vi "Choose Elevator Idle Position.vi"(7 "Hold Low?":bool, 8 "Idle Mode":T1, 10 "Has Trashcan?":bool, 11 "Presets":T2) -> (3 "Pos Out":sgl)   [LabVIEW 2014]
uses:
  Common Code/Elevator Presets.ctl
  Common Code/Elevator Idle Mode.ctl
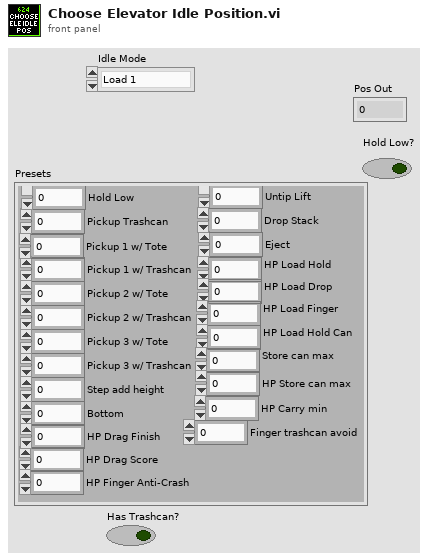
[diagram p1: front panel]
types:
  T1 = typedef "Elevator Idle Mode.ctl" = enum16{"Load 1", "Load 2", "Load 3", "Load Can", "Untip Can", "Step Load", "Drop Stack"}
  T2 = typedef "Elevator Presets.ctl" = cluster{"Pickup 2 w/ Tote":sgl, "Pickup 2 w/ Trashcan":sgl, "Pickup 3 w/ Tote":sgl, "Pickup 3 w/ Trashcan":sgl, "Bottom":sgl, "Pickup 1 w/ Tote":sgl, "Pickup Trashcan":sgl, "Pickup 1 w/ Trashcan":sgl, "Eject":sgl, "Hold Low":sgl, "Step add height":sgl, "Untip Lift":dbl, "Drop Stack":dbl, "HP Load Hold":dbl, "HP Load Drop":dbl, "HP Load Finger":dbl, "HP Load Hold Can":dbl, "Store can max":dbl, "HP Drag Score":dbl, "HP Store can max":dbl, "HP Drag Finish":dbl, "HP Carry min":dbl, "HP Finger Anti-Crash":dbl, "Finger trashcan avoid":dbl}
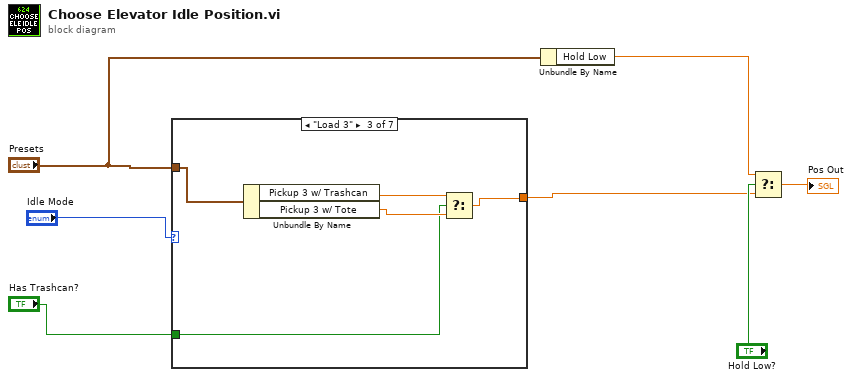
[diagram p0: block diagram]
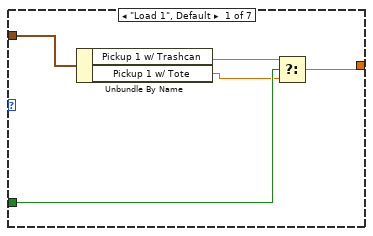
[diagram p2: hidden frame]
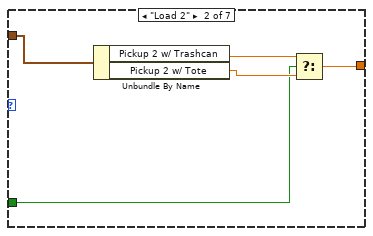
[diagram p3: hidden frame]
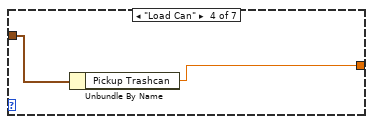
[diagram p4: hidden frame]
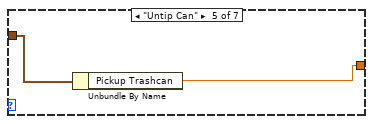
[diagram p5: hidden frame]
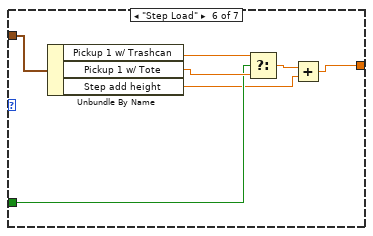
[diagram p6: hidden frame]
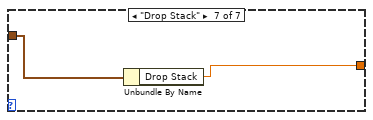
[diagram p7: hidden frame]
diagram:
  n1 = case shown="\"Load 3\"" "Idle Mode" {
    tunnel: "Presets" -> [w12 w14 w18 w24 w26 w31 w35]
    tunnel: "Has Trashcan?" -> [w11 w15 w19 _ _ w30 _]
    tunnel: [w8 w13 w20 w23 w25 w27 w34] -> w1
    frame "Load 1", Default {
      n2 = Unbundle By Name(w12) -> ("Pickup 1 w/ Trashcan"=w10:sgl, "Pickup 1 w/ Tote"=w9:sgl)
      n3 = Select(t=w10, s=w11, f=w9) -> (s? t:f=w8:sgl)
    }
    frame "Load 2" {
      n4 = Unbundle By Name(w14) -> ("Pickup 2 w/ Trashcan"=w17:sgl, "Pickup 2 w/ Tote"=w16:sgl)
      n5 = Select(t=w17, s=w15, f=w16) -> (s? t:f=w13:sgl)
    }
    frame "Load 3" {
      n6 = Unbundle By Name(w18) -> ("Pickup 3 w/ Trashcan"=w21:sgl, "Pickup 3 w/ Tote"=w22:sgl)
      n7 = Select(t=w21, s=w19, f=w22) -> (s? t:f=w20:sgl)
    }
    frame "Load Can" {
      n8 = Unbundle By Name(w24) -> ("Pickup Trashcan"=w23:sgl)
    }
    frame "Untip Can" {
      n9 = Unbundle By Name(w26) -> ("Pickup Trashcan"=w25:sgl)
    }
    frame "Step Load" {
      n10 = Unbundle By Name(w31) -> ("Pickup 1 w/ Trashcan"=w33:sgl, "Pickup 1 w/ Tote"=w32:sgl, "Step add height"=w28:sgl)
      n11 = Select(t=w33, s=w30, f=w32) -> (s? t:f=w29:sgl)
      n12 = Add(x=w29, y=w28) -> (x+y=w27:sgl)
    }
    frame "Drop Stack" {
      n13 = Unbundle By Name(w35) -> ("Drop Stack"=w34:dbl)
    }
  }
  n14 = Unbundle By Name("Presets") -> ("Hold Low"=w6:sgl)
  n15 = Select(t=w6, s="Hold Low?", f=w1) -> (s? t:f=→"Pos Out":dbl)
